vi "Gui_Fill_Laser_Ring.vi"(0 "Refnum Clust":refnum<vi>, 1 "Variant for Path":variant, 3 "error in (no error)":errorcluster) -> (7 "Refnum Clust Out":refnum<vi>, 10 "error out":errorcluster caption="sortie d'erreur")   [LabVIEW 2017]
uses:
  controls/LASER_Inputs.ctl
  controls/EXPERT_Path_Selector.ctl
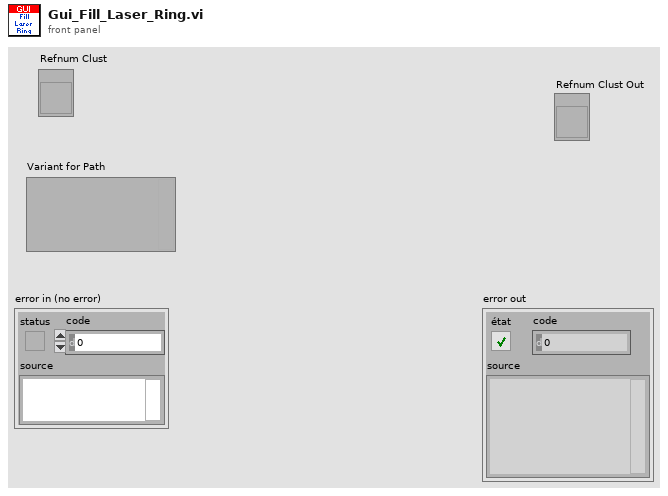
[diagram p1: front panel]
types:
  T1 = typedef "EXPERT_Path_Selector.ctl" = enum16{"Application", "Resources", "Data", "XML", "XML Saved"}
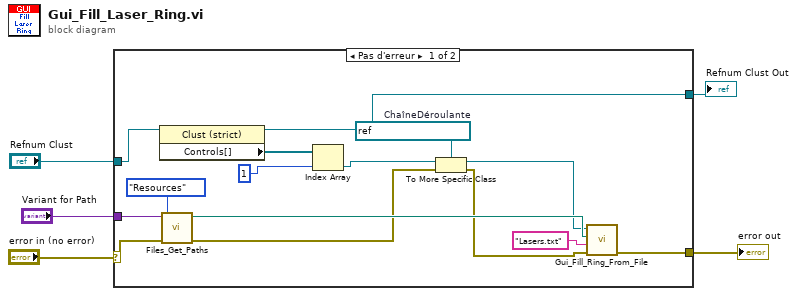
[diagram p0: block diagram]
diagram:
  n1 = case shown="Pas d'erreur" "error in (no error)" {
    selector: "error in (no error)" -> [w19 w22]
    tunnel: [w15 w22] -> w5
    tunnel: "Variant for Path" -> [w20 _]
    tunnel: "Refnum Clust" -> [w13 w21]
    tunnel: [w14 w21] -> w1
    frame No Error {
      w6 = refnum<vi> refnum  # ChaîneDéroulante
      n2 = property class="Clust (strict)"(reference=w13) -> (reference out=w14:refnum<vi>, "Controls[]"=w12:refnum<vi>[])  [unwired: 1 in, 1 out]
      n3 = call "Files_Get_Paths.vi"("error in (no error)"=w19, "EXPERT Path Selector"=EXPERT_Path_Selector."Resources", "Variant"=w20) -> ("error out"=w9:errorcluster, "Path"=w16:path)  [unwired: 7 in]
      n4 = Index Array(array=w12, index=1 ("indice")) -> (element=w10:refnum<vi>)
      n5 = To More Specific Class(target class=w6, reference=w10, error in=w9) -> (specific class reference=w7:refnum<vi>, error out=w8:errorcluster)
      n6 = call "Gui_Fill_Ring_From_File.vi"("error in (no error)"=w8, "Resource Name"="Lasers.txt", "Resource Path"=w16, "Refnum ChneDér"=w7) -> ("error out"=w15:errorcluster)  [unwired: 4 in, 3 out]
    }
    frame Error {
    }
  }
  "error out" <- w5
  "Refnum Clust Out" <- w1
